vi "Keithley_VISA_Read_Write.vi"(8 "error in (no error)":errorcluster, 9 "milliseconds to wait":u32, 10 "command":string, 11 "VISA resource name":refnum<visa-resource-name>) -> (0 "error out":errorcluster, 2 "read buffer":string, 3 "VISA resource name out":refnum<visa-resource-name>)   [LabVIEW 2018]
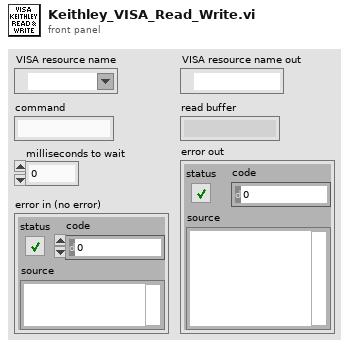
[diagram p1: front panel]
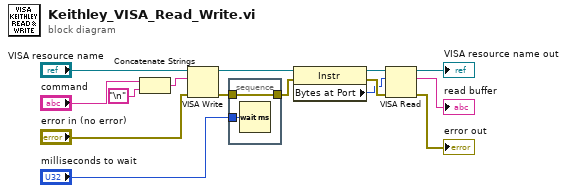
[diagram p0: block diagram]
diagram:
  n1 = Concatenate Strings("command", "\n") -> (w14:string)
  n2 = VISA Write(VISA resource name="VISA resource name", write buffer=w14, error in (no error)="error in (no error)") -> (VISA resource name out=w13:refnum<visa-resource-name>, error out=w9:errorcluster)  [unwired: 1 out]
  n3 = stacked-sequence {
    tunnel: w9 -> [w17]
    tunnel: [w17] -> w8
    tunnel: "milliseconds to wait" -> [w16]
    frame #0 {
      n4 = Wait (ms)(milliseconds to wait=w16) -> ()  [unwired: 1 out]
    }
  }
  n5 = property class="Instr"(reference=w13, error in=w8) -> (reference out=w12:refnum<visa-resource-name>, error out=w11:errorcluster, "Bytes at Port"=w10:u32)
  n6 = VISA Read(VISA resource name=w12, byte count=w10, error in (no error)=w11) -> (VISA resource name out=→"VISA resource name out":refnum<visa-resource-name>, read buffer=→"read buffer":string, error out=→"error out":errorcluster)  [unwired: 1 out]
